vi "Initialize Attributes.vi"(8 "error in (no error)":errorcluster, 10 "Attribute Data":variant, 11 "Example in":refnum<class "Example.lvclass">) -> (0 "error out":errorcluster, 2 "Found?":bool, 3 "Example out":refnum<class "Example.lvclass">)   [LabVIEW 2016, in "CS++Core-Examples.lvlib" / "Example.lvclass"]
doc: "Initialize object attribute.\n\nUnique resources should be allocated elsewhere!"
uses:
  Example.lvclass
  Example.lvclass/Example.ctl
  CSPP_Core/Classes/CS++BaseClasses/Base/CS++Base.lvclass
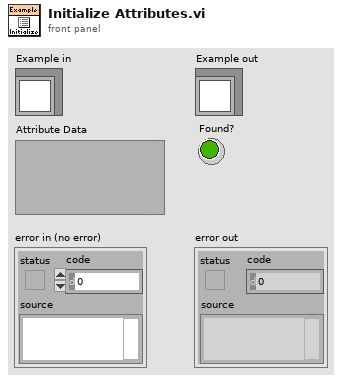
[diagram p1: front panel]
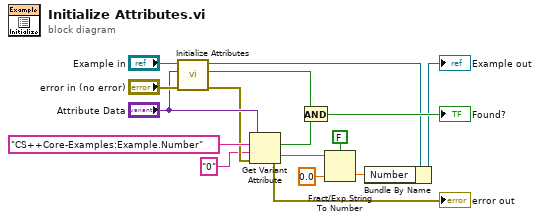
[diagram p0: block diagram]
diagram:
  n1 = call-parent "Initialize Attributes.vi"("error in (no error)"="error in (no error)", "Attribute Data"="Attribute Data", "CS++Base in"="Example in") -> ("error out"=w4:errorcluster, "Found?"=w16:bool, "CS++Base out"=w6:refnum<class "Example.lvclass">)  [unwired: 6 in]
  n2 = Get Variant Attribute(Variant="Attribute Data", name="CS++Core-Examples:Example.Number", default value (empty Variant)="0", error in=w4) -> (found=w11:bool, value=w10:string, error out=→"error out":errorcluster)  [unwired: 1 out]
  n3 = And(x=w16, y=w11) -> (x .and. y?=→"Found?":bool)
  n4 = Fract/Exp String To Number(use system decimal point (T)=FALSE, string=w10, default (0 dbl)=0.0 ("default (0 DBL)")) -> (number=w7:dbl)  [unwired: 1 in, 1 out]
  n5 = Bundle By Name(cluster=w6, "Number"=w7) -> (→"Example out":refnum<class "Example.lvclass">)
